vi "Initialize.vi"(0 "VIPM in":refnum<class "VIP.lvclass">) -> (4 "VIPM out":refnum<class "VIP.lvclass">)   [LabVIEW 2017, in "CL_G3_VIComponentBuilder.lvlib" / "VIP.lvclass"]
doc: "Parses the VIPB for the Product name and Unique name of this VI package."
uses:
  VIP.lvclass
  C:/Tool Chain Support/Software Module Builder/Source/Exports/Exports/Export.lvclass
  Exports/Export.lvclass/Export.ctl
  Exports/Accessors/Write Export Operation Errors.vi
  Exports/Accessors/Read Export Build Specification.vi
  <vilib>/xml/Close Reference(Node).vi
  Exports/Accessors/Write Product Name.vi
  Exports/Accessors/Write unique Name.vi
  Exports/Export.lvclass
  <resource>/objmgr/DOMUserDefRef.rc
  <vilib>/xml/NI_XML.lvlib
  VIPM Utilities/CL_G3_VIPMUtilities.lvlib
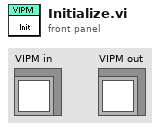
[diagram p1: front panel]
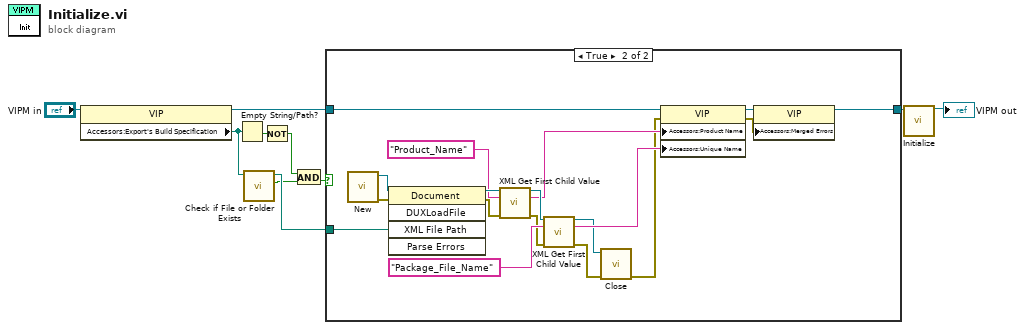
[diagram p0: block diagram]
diagram:
  n1 = property class="VIP"(reference="VIPM in") -> (reference out=w8:refnum<class "VIP.lvclass">, "Accessors:Export's Build Specification"=w5:path)  [unwired: 1 in, 1 out]
  n2 = Empty String/Path?(string/path=w5) -> (empty?=w4:bool)
  n3 = call <vilib>:"Check if File or Folder Exists.vi"("path"=w5) -> ("file or folder exists?"=w3:bool, "dup path"=w6:path)  [unwired: 8 in, 1 out]
  n4 = Not(x=w4) -> (.not. x?=w2:bool)
  n5 = And(x=w2, y=w3) -> (x .and. y?=w1:bool)
  n6 = case shown="True" w1 {
    tunnel: w8 -> [w11 w21]
    tunnel: [w11 w14] -> w7
    tunnel: w6 -> [_ w15]
    frame False {
    }
    frame True {
      n7 = call <vilib>:"New.vi"() -> ("error out"=w28:errorcluster, "DOM document out"=w29:refnum<k20>)  [unwired: 8 in]
      n8 = invoke class="Document" method="DUXLoadFile"(reference=w29, error in=w28, "XML File Path"=w15) -> (reference out=w26:refnum<k20>, error out=w24:errorcluster)  [unwired: 2 in, 3 out]
      n9 = call "XML Get First Child Value.vi"("XML Ref In"=w26, "Tag Name"="Product_Name", "error in (no error)"=w24) -> ("XML Ref Out"=w23:refnum<k20>, "Node Value"=w16:string, "error out"=w22:errorcluster)  [unwired: 10 in]
      n10 = call "XML Get First Child Value.vi"("XML Ref In"=w23, "Tag Name"="Package_File_Name", "error in (no error)"=w22) -> ("XML Ref Out"=w19:refnum<k20>, "Node Value"=w20:string, "error out"=w18:errorcluster)  [unwired: 10 in]
      n11 = call-poly <vilib>:"Close.vi"("error in (no error)"=w18, "node"=w19) -> ("error out"=w13:errorcluster)  [unwired: 7 in]
      n12 = property class="VIP"(reference=w21, error in=w13, "Accessors:Product Name"=w16, "Accessors:Unique Name"=w20) -> (reference out=w17:refnum<class "VIP.lvclass">, error out=w12:errorcluster)
      n13 = property class="VIP"(reference=w17, "Accessors:Merged Errors"=w12) -> (reference out=w14:refnum<class "VIP.lvclass">)  [unwired: 1 in, 1 out]
    }
  }
  n14 = call-parent "Initialize.vi"("Export in"=w7) -> ("Export out"=→"VIPM out":refnum<class "VIP.lvclass">)  [unwired: 14 in]
